vi "Chebyshev Filter (DBL).vi"(0 "init/cont (init:F)":bool, 4 "order":i32=2, 6 "ripple(dB)":dbl=0.1 format="%0.2f", 7 "filter type":T1, 8 "low cutoff freq: fl":dbl=0.125 format="%0.4f", 9 "high cutoff freq: fh":dbl=0.45000000000000007 format="%0.2f", 10 "sampling freq: fs":dbl=1.0 format="%0.2f", 11 "X":dbl[](array[numeric])) -> (1 "error":i32, 3 "Filtered X":dbl[](array[numeric]))   [LabVIEW 2010, in "NI_AALBase.lvlib"]
doc: "Generates a digital Chebyshev filter by calling the Chebyshev Coefficients VI. Wire data to the <B>X</B> input to determine the polymorphic instance to use or manually select the instance."
uses:
  NI_AALBase.lvlib
  Filter Passband Type.ctl
  IIR Cascade Filter (DBL).vi
panel:
  in  "?":dbl[](array[numeric]) format="%0.2f"
  # "Chebyshev Filter"
  # "Filter Controls"
  # "Frequency Controls"
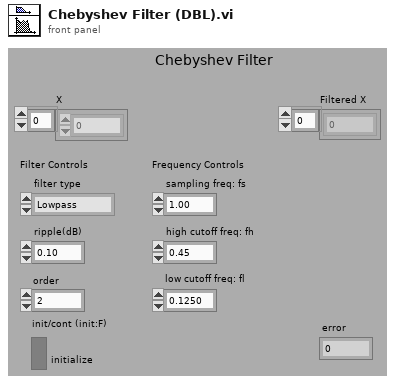
[diagram p1: front panel]
types:
  T1 = typedef "NI_AALBase.lvlib/Filter Passband Type.ctl" = enum32{"Lowpass", "Highpass", "Bandpass", "Bandstop"}
  T2 = cluster{"filter structure":enum32{"IIR 2nd Order", "IIR 4th Order"}, "Reverse Coefficients":dbl[], "Forward Coefficients":dbl[]}
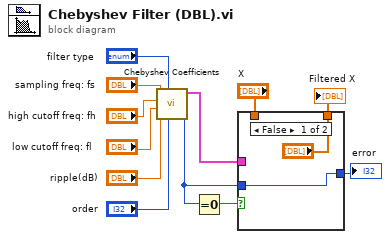
[diagram p0: block diagram]
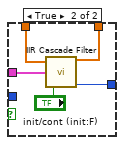
[diagram p2: hidden frame]
diagram:
  n1 = call "Chebyshev Coefficients.vi"("order"="order", "filter type"="filter type", "ripple(dB)"="ripple(dB)", "low cutoff freq: fl"="low cutoff freq: fl", "high cutoff freq: fh"="high cutoff freq: fh", "sampling freq: fs"="sampling freq: fs") -> ("error"=w2:i32, "IIR Filter Cluster"=w1:T2)  [unwired: 4 in]
  n2 = Equal To 0?(x=w2) -> (x = 0?=w3:bool)
  n3 = case shown="False" w3 {
    tunnel: "X" -> [_ w17]
    tunnel: ["?" w18] -> w11
    tunnel: [w13 w19] -> w10
    tunnel: w2 -> [w13 _]
    tunnel: w1 -> [_ w15]
    frame False {
    }
    frame True {
      n4 = call-poly "IIR Cascade Filter.vi"("init/cont (init:F)"="init/cont (init:F)", "IIR Filter Cluster"=w15, "X"=w17) -> ("error"=w19:i32, "Filtered X"=w18:dbl[])
    }
  }
  "Filtered X" <- w11
  "error" <- w10
